vi "Configure Measurement (Phase).vi"(8 "error in (no error)":errorcluster, 9 "Phase Reference Channel (2:Channel 2)":i32(ring)=2 items=["Channel 1"=1, "Channel 2"=2], 10 "Phase Input Channel (1:Channel 1)":i32(ring)=1 items=["Channel 1"=1, "Channel 2"=2], 11 "VISA resource name":refnum<visa-resource-name>) -> (0 "error out":errorcluster, 3 "VISA resource name out":refnum<visa-resource-name>)   [LabVIEW 2024, in "Agilent 532XX Series.lvlib"]
doc: "Configures the settings required for a Phase measurement.\n\n<B>Note:</B> This VI only applies to the Agilent 53220A/53230A."
uses:
  Agilent 532XX Series.lvlib
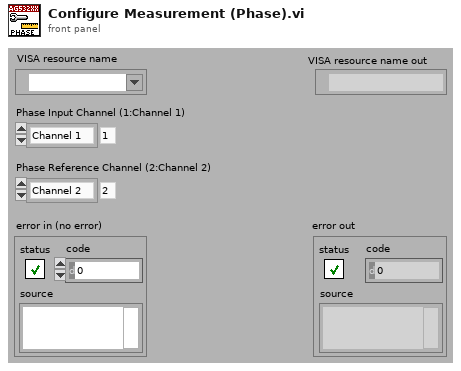
[diagram p1: front panel]
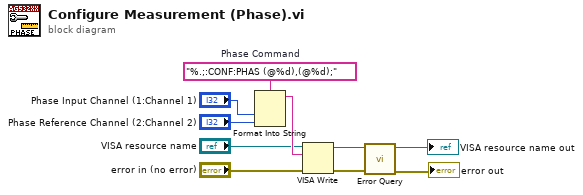
[diagram p0: block diagram]
diagram:
  w10 = "%.;:CONF:PHAS (@%d),(@%d);"  # Phase Command
  n1 = Format Into String(format string=w10, "Phase Input Channel (1:Channel 1)", "Phase Reference Channel (2:Channel 2)") -> (resulting string=w4:string)  [unwired: 2 in, 1 out]
  n2 = VISA Write(VISA resource name="VISA resource name", write buffer=w4, error in (no error)="error in (no error)") -> (VISA resource name out=w5:refnum<visa-resource-name>, error out=w7:errorcluster)  [unwired: 1 out]
  n3 = call "Error Query.vi"("error in (no error)"=w7, "VISA resource name"=w5) -> ("error out"=→"error out":errorcluster, "VISA resource name out"=→"VISA resource name out":refnum<visa-resource-name>)  [unwired: 8 out]
